vi "AFMnoisedensityFit.vi"() -> ()   [LabVIEW 2010]
uses:
  <vilib>/gmath/NumericalOptimization/Nonlinear Curve Fit LM formula string.vi
  <vilib>/gmath/NumericalOptimization/Nonlinear Curve Fit LM bound.vi
  <userlib>/Nanonis Prog Interface V5/Nanonis Prog Interface.lvlib
  <vilib>/gmath/NI_Gmath.lvlib
panel:
  in  "Curve BW(Hz)":dbl=40.0
  in  "Fitting Weight (only for filter corection)":dbl[](array[numeric])=[1.0, 1.0, 5.0, 50.0, 0.1]
  in  "Filter\nCorrection":bool
  out "n_q from fit (fm/sqrt(Hz))":dbl format="%#_5e"
  out "Sens from fit (uV/pm)":dbl format="%#_5e"
  out "V_th from fit  (uV)":dbl format="%#_5e"
  out "n_q (fm/sqrt(Hz))":dbl format="%#_5e"
  out "Sensitivity (uV/pm)":dbl format="%#_5e"
  out "V_th (uV)":dbl format="%#_5e"
  in  "Bandwidth (Hz)":dbl=48.75
  out "alpha_th (fm/sqrt(Hz)":dbl format="%#_5e"
  out "A_th (fm)":dbl format="%#_5e"
  in  "k (N/m)":dbl=1800.0
  in  "Temperature (K)":dbl=300.0
  out "Noise density (nV/sqrt(Hz))":dbl format="%#_5e"
  out "Cernter Freq(Hz)":dbl
  out "Cernter Freq(dF)":dbl
  out "Q factor":dbl format="%#_5f"
  in  "initial dF(Hz)":dbl=20.0
  in  "Start Fitting":bool
  out "Waveform Graph":cluster{"f0":dbl, "df":dbl, dbl[][]}(graph)
  in  "Filter Order\n(0=no change)":u32=1 max=8 step=1
  in  "Weighting Mode":enum16{"no change", "Linear", "Exponential"}(ring)
  in  "Averaging mode":T1(ring)
  in  "Average Count":u32=1 min=1
  in  "Center Frequency(Hz)":dbl=32800.0
  in  "Filter Cutoff(Hz)":dbl=389.0
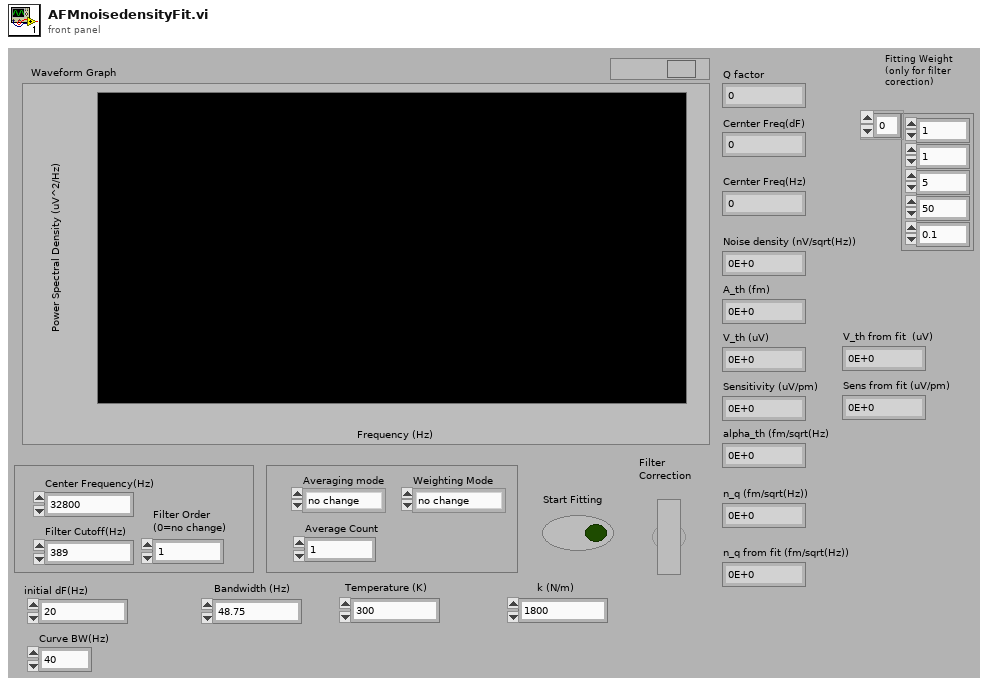
[diagram p1: front panel]
types:
  T1 = enum16{"no change", "None", "Vector", "RMS", "Peak hold"}
  T2 = enum8{"Enabled", "Disabled", "Disabled and Grayed Out"}
  T3 = cluster{"model":string, "Parameters":string[], "x":string}
  T4 = cluster{"Averaging mode":enum16{"no change", "None", "Vector", "RMS", "Peak hold"}, "Weighting Mode":enum16{"no change", "Linear", "Exponential"}, "Average Count":u32}
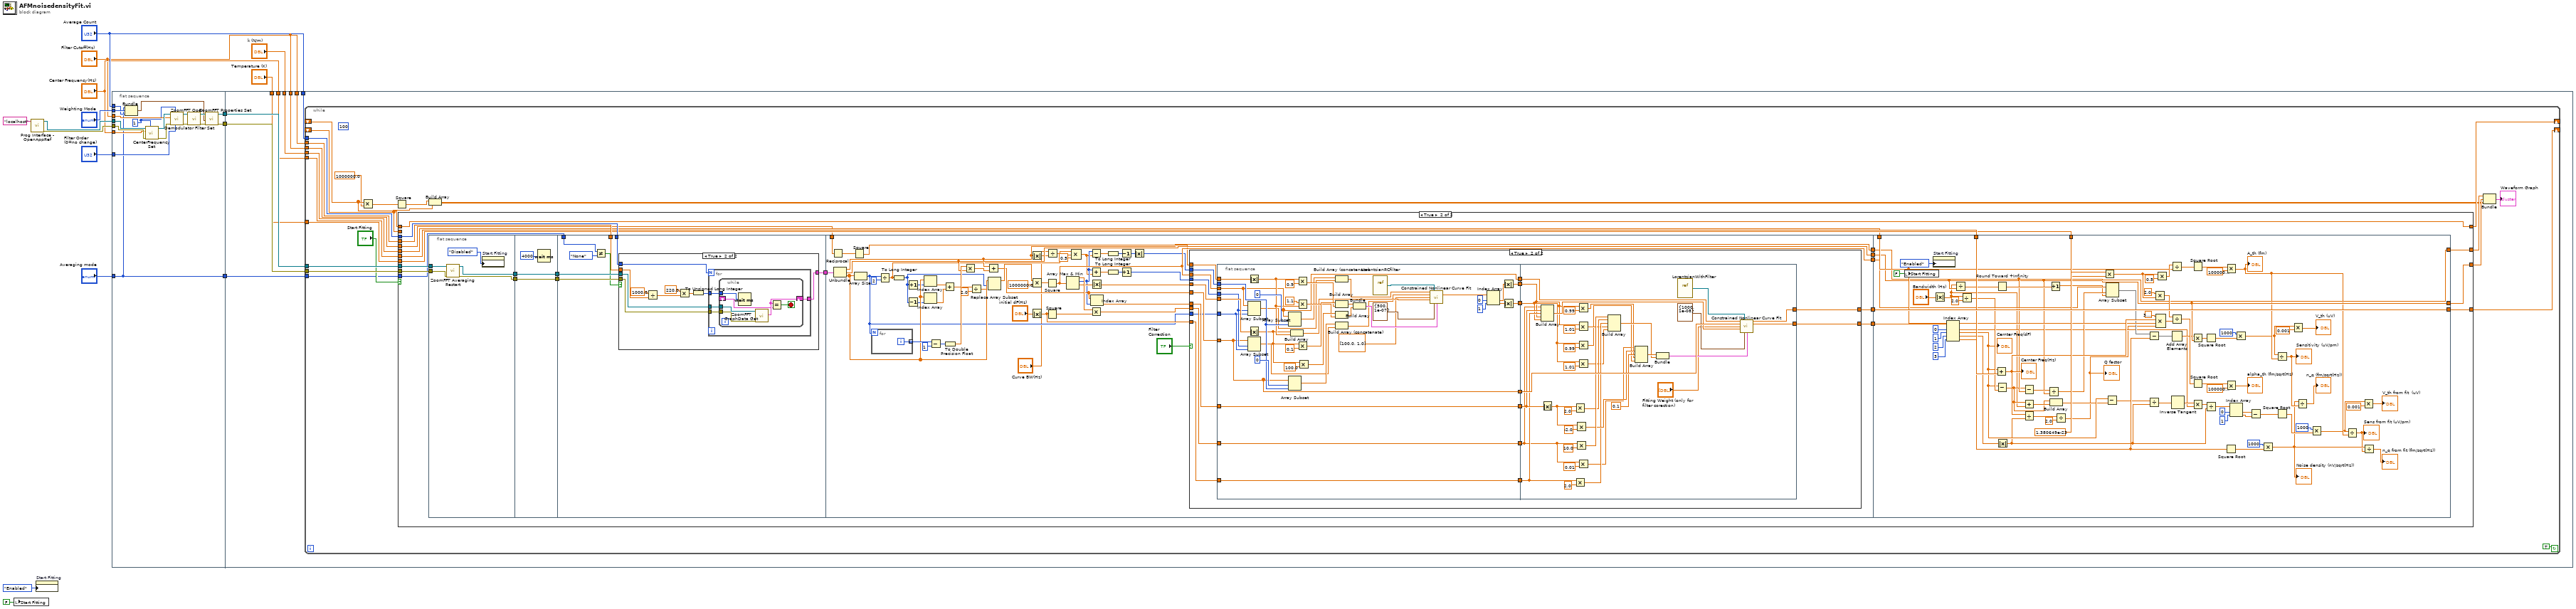
[diagram p0: block diagram]
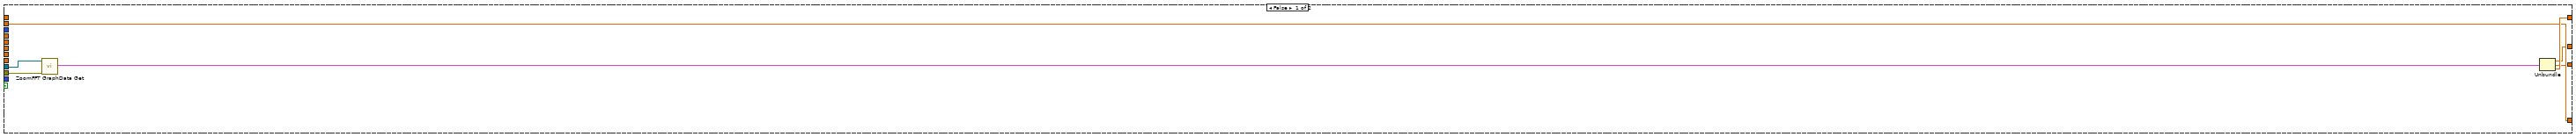
[diagram p2: hidden frame]
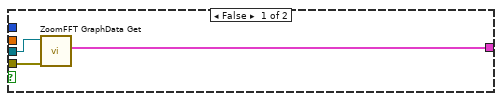
[diagram p3: hidden frame]
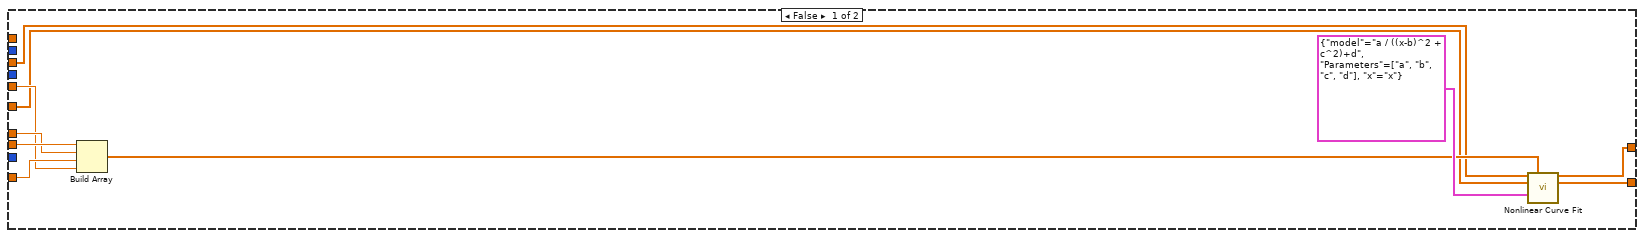
[diagram p4: hidden frame]
diagram:
  n1 = local write "Start Fitting"(FALSE) -> ()
  n2 = call <userlib>:"Prog Interface - OpenAppRef.vi"("Machine name (local machine IP)"="localhost" ("machine name (localhost)")) -> ("Error out"=w13:errorcluster, "Application reference"=w15:refnum<vi>)  [unwired: 5 in]
  n3 = property on="Start Fitting" class="Bool (strict)"("DisabledEnum"=T2."Enabled" ("Disabled")) -> ()  [unwired: 2 in, 2 out]
  n4 = flat-sequence {
    tunnel: w15 -> [w28]
    tunnel: [w34] -> w14
    tunnel: w13 -> [w27]
    tunnel: "Average Count" -> [w29]
    tunnel: "Averaging mode" -> [w17]
    tunnel: "Weighting Mode" -> [w30]
    tunnel: "Center Frequency(Hz)" -> [w26]
    tunnel: "Filter Cutoff(Hz)" -> [w21]
    tunnel: "Filter Order\n(0=no change)" -> [w20]
    tunnel: [w18] -> w9
    tunnel: [w17] -> w6
    tunnel: w14 -> [w43]
    tunnel: w9 -> [w42]
    tunnel: "Average Count" -> [w41]
    tunnel: "Filter Cutoff(Hz)" -> [w40]
    tunnel: w6 -> [w39]
    tunnel: "Center Frequency(Hz)" -> [w38]
    tunnel: "Temperature (K)" -> [w37]
    tunnel: "k (N/m)" -> [w36]
    tunnel: "Filter Cutoff(Hz)" -> [w35]
    frame #0 {
      w19 = 1
      n5 = Bundle("Averaging mode"=w17, "Weighting Mode"=w30, "Average Count"=w29) -> (w31:T4)  [unwired: 1 in]
      n6 = call <userlib>:"CenterFrequency Set.vi"("Modulator index"=w19, "Error in (no error)"=w27, "Center Frequency (Hz)"=w26, "Application ref in"=w28) -> ("Error out"=w22:errorcluster, "Application ref out"=w25:refnum<vi>)  [unwired: 6 in]
      n7 = call <userlib>:"Demodulator Filter Set.vi"("Filter Order (1...8) (0=no change)"=w20, "Demodulator index"=w19, "Error in"=w22, "Cutoff Frq (Hz) (0=no change)"=w21, "Application ref in"=w25) -> ("Error out"=w23:errorcluster, "Application ref out"=w24:refnum<vi>)  [unwired: 5 in]
      n8 = call <userlib>:"ZoomFFT Open.vi"("Error in (no error)"=w23, "Application ref in"=w24) -> ("Error out"=w32:errorcluster, "Application ref out"=w33:refnum<vi>)  [unwired: 8 in]
      n9 = call <userlib>:"ZoomFFT Properties Set.vi"("Error in (no error)"=w32, "Averaging"=w31, "Application ref in"=w33) -> ("Error out"=w18:errorcluster, "Application ref out"=w34:refnum<vi>)  [unwired: 5 in]
    }
    frame #1 {
      n10 = while {
        tunnel: w43 -> [w65]
        tunnel: w42 -> [w64]
        tunnel: w41 -> [w50]
        tunnel: w40 -> [w61]
        shift-right: [w59] -> _
        shift-left: _ -> [w44]
        shift-right: [w60] -> _
        shift-left: _ -> [w52]
        tunnel: w39 -> [w55]
        tunnel: w38 -> [w49]
        tunnel: w37 -> [w48]
        tunnel: w36 -> [w47]
        tunnel: w35 -> [w46]
        stop <- TRUE continue-if-true
        (unwired) 100
        n11 = Multiply(x=w52, y=1000000.0) -> (x*y=w53:dbl[])
        n12 = Square(x=w53) -> (x^2=w45:dbl[])
        n13 = case shown="True" "Start Fitting" {
          tunnel: w65 -> [w72 w95]
          tunnel: w64 -> [w71 w94]
          tunnel: w61 -> [_ w89]
          tunnel: [w69 w84] -> w60
          tunnel: [w68 w85] -> w59
          tunnel: w52 -> [_ w84]
          tunnel: w44 -> [w68 _]
          tunnel: [w67 w83] -> w58
          tunnel: [w66 w82] -> w57
          tunnel: w55 -> [_ w81]
          tunnel: w50 -> [_ w79]
          tunnel: w49 -> [_ w77]
          tunnel: w48 -> [_ w76]
          tunnel: w47 -> [_ w75]
          tunnel: w46 -> [_ w73]
          frame False {
            n14 = call <userlib>:"ZoomFFT GraphData Get.vi"("Error in (no error)"=w71, "Application ref in"=w72) -> ("Spectrum data"=w70:cluster{"f0":dbl, "df":dbl, "values":dbl[]})  [unwired: 7 in, 2 out]
            n15 = Unbundle(w70) -> ("f0"=w67:dbl, "df"=w66:dbl, "values"=w69:dbl[])
          }
          frame True {
            n16 = flat-sequence {
              tunnel: [w100] -> w93
              tunnel: [w99] -> w91
              tunnel: w94 -> [w96]
              tunnel: w95 -> [w97]
              tunnel: w93 -> [w103]
              tunnel: [w103] -> w92
              tunnel: w91 -> [w102]
              tunnel: [w102] -> w90
              tunnel: w92 -> [w111]
              tunnel: w90 -> [w110]
              tunnel: w89 -> [w109]
              tunnel: [w108] -> w88
              tunnel: w81 -> [w106]
              tunnel: w79 -> [w104]
              tunnel: w88 -> [w181]
              tunnel: [w152] -> w87
              tunnel: [w162] -> w86
              tunnel: [w165] -> w80
              tunnel: [w164] -> w78
              tunnel: [w163] -> w74
              tunnel: w73 -> [w155]
              tunnel: w87 -> [w344]
              tunnel: w86 -> [w337]
              tunnel: [w374] -> w85
              tunnel: [w344] -> w83
              tunnel: [w337] -> w82
              tunnel: w80 -> [w374]
              tunnel: w78 -> [w369]
              tunnel: w77 -> [w368]
              tunnel: w76 -> [w366]
              tunnel: w75 -> [w356]
              tunnel: w74 -> [w347]
              frame #0 {
                n17 = call <userlib>:"ZoomFFT Averaging Restart.vi"("Error in (no error)"=w96, "Application ref in"=w97) -> ("Error out"=w99:errorcluster, "Application ref out"=w100:refnum<vi>)  [unwired: 8 in]
                n18 = property on="Start Fitting" class="Bool (strict)"("DisabledEnum"=T2."Disabled" ("Disabled")) -> ()  [unwired: 2 in, 2 out]
              }
              frame #1 {
                n19 = Wait (ms)(milliseconds to wait=4000) -> ()  [unwired: 1 out]
              }
              frame #2 {
                n20 = Not Equal?(x=w106, y=T1."None") -> (x != y?=w107:bool)
                n21 = case shown="True" w107 {
                  tunnel: w111 -> [w113 w121]
                  tunnel: w110 -> [w112 w122]
                  tunnel: w109 -> [_ w124]
                  tunnel: [w114 w123] -> w108
                  tunnel: w104 -> [_ w115]
                  frame False {
                    n22 = call <userlib>:"ZoomFFT GraphData Get.vi"("Error in (no error)"=w112, "Application ref in"=w113) -> ("Spectrum data"=w114:cluster{"f0":dbl, "df":dbl, "values":dbl[]})  [unwired: 7 in, 2 out]
                  }
                  frame True {
                    n23 = Divide(x=1000.0, y=w124) -> (x/y=w118:dbl)
                    n24 = Multiply(x=220.0, y=w118) -> (x*y=w117:dbl)
                    n25 = To Unsigned Long Integer(number=w117) -> (unsigned 32bit integer=w116:u32)
                    n26 = for {
                      N: w115 -> [_]
                      tunnel: [w128] -> w123
                      tunnel: w122 -> [w127]
                      tunnel: w121 -> [w126]
                      tunnel: w116 -> [w125]
                      n27 = while {
                        tunnel: w126 -> [w134]
                        shift-right: [w131] -> w128
                        shift-left: _ -> [w130]
                        tunnel: w127 -> [w133]
                        tunnel: w125 -> [w129]
                        stop <- w132 stop-if-true
                        n28 = Wait (ms)(milliseconds to wait=w129) -> ()  [unwired: 1 out]
                        n29 = call <userlib>:"ZoomFFT GraphData Get.vi"("Error in (no error)"=w133, "Application ref in"=w134) -> ("Spectrum data"=w131:cluster{"f0":dbl, "df":dbl, "values":dbl[]})  [unwired: 7 in, 2 out]
                        n30 = Equal?(x=w131, y=w130) -> (x = y?=w132:bool)
                      }
                    }
                  }
                }
              }
              frame #3 {
                n31 = Reciprocal(x=w155) -> (1/x=w154:dbl)
                n32 = Unbundle(w181) -> ("f0"=w152:dbl, "df"=w162:dbl, "values"=w169:dbl[])
                n33 = Square(x=w154) -> (x^2=w153:dbl)
                n34 = Array Size(array=w169) -> (size(s)=w137:i32)
                n35 = for {
                  N: w137 -> [_]
                  tunnel: [w294] -> w186 mode=indexing
                  i -> [w294]
                }
                n36 = Divide(x=w137, y=2) -> (x/y=w146:dbl)
                n37 = To Long Integer(number=w146) -> (32bit integer=w156:i32)
                n38 = Increment(x=w156) -> (x+1=w158:i32)
                n39 = Decrement(x=w156) -> (x-1=w157:i32)
                n40 = Index Array(array=w169, index=w158) -> (element=w171:dbl)
                n41 = Index Array(array=w169, index=w157) -> (element=w170:dbl)
                n42 = Subtract(x=w186, y=1) -> (x-y=w184:i32[])
                n43 = Add(x=w171, y=w170) -> (x+y=w168:dbl)
                n44 = To Double Precision Float(number=w184) -> (double precision float=w183:dbl[])
                n45 = Multiply(x=w183, y=w162) -> (x*y=w182:dbl[])
                n46 = Divide(x=w168, y=2.0) -> (x/y=w160:dbl)
                n47 = Add(x=w152, y=w182) -> (x+y=w166:dbl[])
                n48 = Replace Array Subset(array=w169, new element=w160, index=w156) -> (w172:dbl[])
                n49 = Absolute Value(x=w152) -> (abs(x)=w150:dbl)
                n50 = Multiply(x=w172, y=1000000.0) -> (x*y=w176:dbl[])
                n51 = Absolute Value(x="initial dF(Hz)") -> (abs(x)=w151:dbl)
                n52 = Square(x=w176) -> (x^2=w163:dbl[])
                n53 = Square(x=w151) -> (x^2=w178:dbl)
                n54 = Divide(x="Curve BW(Hz)", y=w150) -> (x/y=w147:dbl)
                n55 = Array Max & Min(array=w163) -> (max value=w179:dbl, max index (indices)=w140:i32, min value=w159:dbl)  [unwired: 1 out]
                n56 = Compound Arithmetic op=MULTIPLY(w147, w146, 0.5 ("value")) -> (w139:dbl)
                n57 = Subtract(x=w140, y=w139) -> (x-y=w149:dbl)
                n58 = Add(x=w140, y=w139) -> (x+y=w138:dbl)
                n59 = Multiply(x=w179, y=w178) -> (x*y=w180:dbl)
                n60 = Absolute Value(x=w159) -> (abs(x)=w143:dbl)
                n61 = Index Array(array=w166, index=w140) -> (element=w177:dbl)
                n62 = To Long Integer(number=w149) -> (32bit integer=w148:i32)
                n63 = To Long Integer(number=w138) -> (32bit integer=w142:i32)
                n64 = Decrement(x=w148) -> (x-1=w145:i32)
                n65 = Increment(x=w142) -> (x+1=w141:i32)
                n66 = Absolute Value(x=w145) -> (abs(x)=w144:i32)
                n67 = case shown="True" "Filter\nCorrection" {
                  tunnel: w180 -> [w193 w207]
                  tunnel: w143 -> [w190 w208]
                  tunnel: w177 -> [w191 w211]
                  tunnel: w151 -> [w192 w210]
                  tunnel: w166 -> [w189 w214]
                  tunnel: [w188 w213] -> w165
                  tunnel: [w187 w212] -> w164
                  tunnel: w163 -> [w194 w215]
                  tunnel: w153 -> [_ w209]
                  tunnel: w144 -> [_ w199]
                  tunnel: w141 -> [_ w198]
                  tunnel: w137 -> [_ w197]
                  frame False {
                    n68 = Build Array(w193, w191, w192, w190) -> (w195:dbl[])
                    n69 = call-poly <vilib>:"Nonlinear Curve Fit.vi"("Y"=w194, "initial parameters"=w195, "X"=w189, "model description"=T3 {"model"="a / ((x-b)^2 + c^2)+d", "Parameters"=["a", "b", "c", "d"], "x"="x"}) -> ("best nonlinear fit"=w188:dbl[], "best fit parameters"=w187:dbl[])  [unwired: 7 in, 3 out]
                  }
                  frame True {
                    n70 = flat-sequence {
                      tunnel: w207 -> [w255]
                      tunnel: w208 -> [w229]
                      tunnel: w209 -> [w231]
                      tunnel: w210 -> [w256]
                      tunnel: w211 -> [w257]
                      tunnel: w214 -> [w224]
                      tunnel: w215 -> [w227]
                      tunnel: [w227] -> w206
                      tunnel: [w224] -> w205
                      tunnel: [w257] -> w204
                      tunnel: [w256] -> w203
                      tunnel: [w247] -> w202
                      tunnel: [w250] -> w201
                      tunnel: [w255] -> w200
                      tunnel: w199 -> [w246]
                      tunnel: w198 -> [w226]
                      tunnel: w197 -> [w225]
                      tunnel: [w258] -> w213
                      tunnel: [w290] -> w212
                      tunnel: w206 -> [w293]
                      tunnel: w205 -> [w292]
                      tunnel: w204 -> [w279]
                      tunnel: w203 -> [w275]
                      tunnel: w202 -> [w268]
                      tunnel: w201 -> [w264]
                      tunnel: w200 -> [w260]
                      frame #0 {
                        n71 = Array Subset(array=w227, index=w226, length=w225) -> (w222:dbl[])
                        n72 = Array Subset(array=w224, index=w226, length=w225) -> (w219:dbl[])
                        n73 = Absolute Value(x=w231) -> (abs(x)=w230:dbl)
                        n74 = Absolute Value(x=w229) -> (abs(x)=w228:dbl)
                        n75 = Array Subset(array=w227, index=0, length=w246) -> (w223:dbl[])
                        n76 = Array Subset(array=w224, index=0, length=w246) -> (w220:dbl[])
                        n77 = Build Array(w228, w230) -> (w218:dbl[])
                        n78 = Multiply(x=w230, y=0.9) -> (x*y=w240:dbl)
                        n79 = Multiply(x=1.1, y=w230) -> (x*y=w238:dbl)
                        n80 = Multiply(x=w228, y=0.1) -> (x*y=w241:dbl)
                        n81 = Multiply(x=w228, y=100.0) -> (x*y=w239:dbl)
                        n82 = Build Array (concatenate)(w223, w222) -> (w221:dbl[])
                        n83 = Build Array(w241, w240) -> (w243:dbl[])
                        n84 = Build Array(w239, w238) -> (w242:dbl[])
                        n85 = Build Array (concatenate)(w220, w219) -> (w217:dbl[])
                        n86 = Bundle(w243, w242) -> (w233:cluster{dbl[], dbl[]})  [unwired: 1 in]
                        n87 = vi-ref "LorentzianRCfilter.vi"() -> (w244:refnum<vi>)
                        n88 = call-poly <vilib>:"Constrained Nonlinear Curve Fit.vi"("Y"=w221, "f(x,a)"=w244, "X"=w217, "Weight"=dbl[] [100.0, 1.0], "initial parameters"=w218, "termination"=cluster{"max iteration":i32, "tolerance":dbl} {"max iteration"=500, "tolerance"=1e-07}, "parameter bounds"=w233) -> ("best fit parameters"=w245:dbl[])  [unwired: 3 in, 5 out]
                        n89 = Index Array(array=w245, index #1=0 ("index"), index #2=1 ("index")) -> (element #1=w249:dbl, element #2=w248:dbl)
                        n90 = Absolute Value(x=w249) -> (abs(x)=w250:dbl)
                        n91 = Absolute Value(x=w248) -> (abs(x)=w247:dbl)
                      }
                      frame #1 {
                        n92 = Build Array(w260, w279, w275, w264, w268) -> (w291:dbl[])
                        n93 = Absolute Value(x=w279) -> (abs(x)=w278:dbl)
                        n94 = Multiply(x=w278, y=2.0) -> (x*y=w280:dbl)
                        n95 = Multiply(x=w275, y=2.0) -> (x*y=w276:dbl)
                        n96 = Multiply(x=w278, y=-2.0) -> (x*y=w282:dbl)
                        n97 = Multiply(x=w260, y=10.0) -> (x*y=w284:dbl)
                        n98 = Multiply(x=w264, y=0.99) -> (x*y=w265:dbl)
                        n99 = Multiply(x=w264, y=1.01) -> (x*y=w273:dbl)
                        n100 = Multiply(x=w268, y=0.99) -> (x*y=w270:dbl)
                        n101 = Multiply(x=w268, y=1.01) -> (x*y=w267:dbl)
                        n102 = Multiply(x=w260, y=0.01) -> (x*y=w262:dbl)
                        n103 = Build Array(w284, w280, w276, w273, w267) -> (w285:dbl[])
                        n104 = Build Array(w262, w282, 0.1 ("element"), w265, w270) -> (w286:dbl[])
                        n105 = Bundle(w286, w285) -> (w271:cluster{dbl[], dbl[]})  [unwired: 1 in]
                        n106 = vi-ref "LorentzianWithFilter.vi"() -> (w289:refnum<vi>)
                        n107 = call-poly <vilib>:"Constrained Nonlinear Curve Fit.vi"("Y"=w293, "f(x,a)"=w289, "X"=w292, "Weight"="Fitting Weight (only for filter corection)", "initial parameters"=w291, "termination"=cluster{"max iteration":i32, "tolerance":dbl} {"max iteration"=1000, "tolerance"=1e-08}, "parameter bounds"=w271) -> ("best nonlinear fit"=w258:dbl[], "best fit parameters"=w290:dbl[])  [unwired: 3 in, 4 out]
                      }
                    }
                  }
                }
              }
              frame #4 {
                n108 = local write "Start Fitting"(FALSE) -> ()
                n109 = property on="Start Fitting" class="Bool (strict)"("DisabledEnum"=T2."Enabled" ("Disabled")) -> ()  [unwired: 2 in, 2 out]
                n110 = Absolute Value(x="Bandwidth (Hz)") -> (abs(x)=w318:dbl)
                n111 = Index Array(array=w369, index #1=0 ("index"), index #2=1 ("index"), index #3=2 ("index"), index #4=3 ("index")) -> (element #1=w326:dbl, element #2=w322:dbl, element #3=w305:dbl, element #4=w335:dbl)
                "Cernter Freq(dF)" <- w322
                n112 = Divide(x=w318, y=w337) -> (x/y=w346:dbl)
                n113 = Divide(x=w318, y=2.0) -> (x/y=w342:dbl)
                n114 = Add(x=w322, y=w368) -> (x+y=w357:dbl)
                "Cernter Freq(Hz)" <- w357
                n115 = Round Toward +Infinity(x=w346) -> (ceil(x): smallest int >= x=w345:dbl)
                n116 = Subtract(x=w322, y=w342) -> (x-y=w319:dbl)
                n117 = Absolute Value(x=w305) -> (abs(x)=w304:dbl)
                n118 = Subtract(x=w319, y=w344) -> (x-y=w343:dbl)
                n119 = Add(x=w319, y=w318) -> (x+y=w320:dbl)
                n120 = Divide(x=w357, y=w304) -> (x/y=w303:dbl)
                n121 = Divide(x=w343, y=w337) -> (x/y=w339:dbl)
                n122 = Increment(x=w345) -> (x+1=w338:dbl)
                n123 = Build Array(w319, w320) -> (w321:dbl[])
                n124 = Divide(x=w303, y=2.0) -> (x/y=w302:dbl)
                "Q factor" <- w302
                n125 = Multiply(x=1.380649e-23, y=w366) -> (x*y=w359:dbl)
                n126 = Subtract(x=w322, y=w321) -> (x-y=w324:dbl[])
                n127 = Array Subset(array=w347, index=w339, length=w338) -> (w336:dbl[])
                n128 = Subtract(x=w336, y=w335) -> (x-y=w334:dbl[])
                n129 = Divide(x=w324, y=w304) -> (x/y=w325:dbl[])
                n130 = Multiply(x=2.0, y=w359) -> (x*y=w355:dbl)
                n131 = Multiply(x=w359, y=0.5) -> (x*y=w364:dbl)
                n132 = Compound Arithmetic op=MULTIPLY(3.141592653589793, w357, w356, w302) -> (w354:dbl)
                n133 = Divide(x=w364, y=w356) -> (x/y=w365:dbl)
                n134 = Divide(x=w355, y=w354) -> (x/y=w353:dbl)
                n135 = Add Array Elements(numeric array=w334) -> (sum=w333:dbl)
                n136 = Inverse Tangent(1:w325) -> (0:w327:dbl[])
                n137 = Square Root(x=w365) -> (sqrt(x)=w352:dbl)
                n138 = Multiply(x=w333, y=w337) -> (x*y=w332:dbl)
                n139 = Square Root(x=w353) -> (sqrt(x)=w350:dbl)
                n140 = Multiply(x=w327, y=w326) -> (x*y=w323:dbl[])
                n141 = Square Root(x=w332) -> (sqrt(x)=w330:dbl)
                n142 = Divide(x=w323, y=w304) -> (x/y=w317:dbl[])
                n143 = Square Root(x=w335) -> (sqrt(x)=w362:dbl)
                n144 = Multiply(x=w352, y=1000000000000000.0) -> (x*y=w309:dbl)
                "A_th (fm)" <- w309
                n145 = Multiply(x=w350, y=1000000000000000.0) -> (x*y=→"alpha_th (fm/sqrt(Hz)":dbl)
                n146 = Index Array(array=w317, index #1=0 ("index"), index #2=1 ("index")) -> (element #1=w314:dbl, element #2=w313:dbl)
                n147 = Multiply(x=1000, y=w330) -> (x*y=w300:dbl)
                n148 = Subtract(x=w314, y=w313) -> (x-y=w310:dbl)
                n149 = Multiply(x=1000, y=w362) -> (x*y=w307:dbl)
                "Noise density (nV/sqrt(Hz))" <- w307
                n150 = Divide(x=w300, y=w309) -> (x/y=w328:dbl)
                "Sensitivity (uV/pm)" <- w328
                n151 = Square Root(x=w310) -> (sqrt(x)=w311:dbl)
                n152 = Multiply(x=w300, y=0.001) -> (x*y=→"V_th (uV)":dbl)
                n153 = Divide(x=w307, y=w328) -> (x/y=→"n_q (fm/sqrt(Hz))":dbl)
                n154 = Multiply(x=1000, y=w311) -> (x*y=w296:dbl)
                n155 = Divide(x=w296, y=w309) -> (x/y=w306:dbl)
                "Sens from fit (uV/pm)" <- w306
                n156 = Multiply(x=w296, y=0.001) -> (x*y=→"V_th from fit  (uV)":dbl)
                n157 = Divide(x=w307, y=w306) -> (x/y=→"n_q from fit (fm/sqrt(Hz))":dbl)
              }
            }
          }
        }
        n158 = Build Array(w45, w44) -> (w54:dbl[][])
        n159 = Bundle("f0"=w58, "df"=w57, w54) -> (→"Waveform Graph":cluster{"f0":dbl, "df":dbl, dbl[][]})  [unwired: 1 in]
      }
    }
  }
